vi "WPI_I2CVerifyString.vi"(8 "error in (no error)":errorcluster, 9 "Expected":string, 10 "Register Address":u8, 11 "I2CDevRef":T1={"DevStatus"={"status"=FALSE, "code"=0, "source"=""}, "Device Address"=0, "Handle"=0, "I2C Bus"=enum."Invalid"} {"Device Address" format="%.0x"}) -> (0 "error out":errorcluster, 3 "I2CDevRef":T1={"DevStatus"={"status"=FALSE, "code"=0, "source"=""}, "Device Address"=0, "Handle"=0, "I2C Bus"=enum."Invalid"} {"Device Address" format="%.0x"})   [LabVIEW 2017]
doc: "Reads consecutive registers from the I2C sensor you specify and compares the register strings to an expected value. This VI returns an error if the register strings do not match.\n\nThis software is licensed. Open the labview\\readme\\WPI Robotics Library Open Source License.txt file for more information."
uses:
  <vilib>/Rock Robotics/WPI/I2C/WPI_I2CDevRef.ctl
  <vilib>/Rock Robotics/SystemInterfaces/i2clib/i2c_bus.ctl
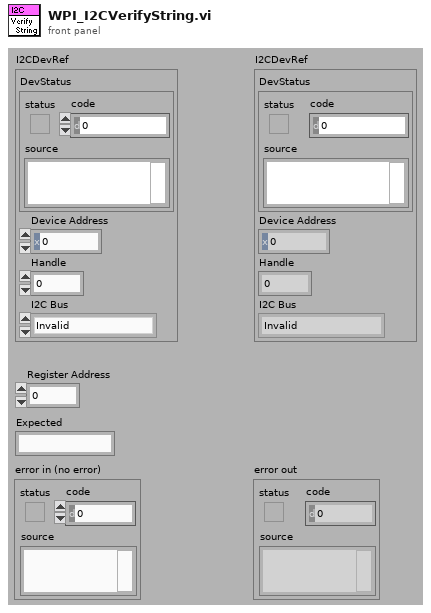
[diagram p1: front panel]
types:
  T1 = typedef "WPI_I2CDevRef.ctl" = cluster{"DevStatus":errorcluster, "Device Address":u8, "Handle":i32, "I2C Bus":T2}
  T2 = typedef "i2c_bus.ctl" = enum16{"I2C On-Board", "I2C MXP", "Invalid"}
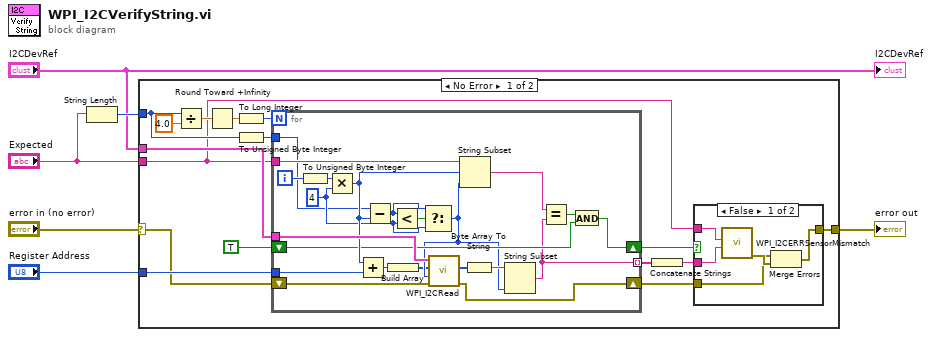
[diagram p0: block diagram]
diagram:
  n1 = String Length(string="Expected") -> (length=w5:i32)
  n2 = case shown="No Error" "error in (no error)" {
    selector: "error in (no error)" -> [w15 w51]
    tunnel: w5 -> [w11 _]
    tunnel: [w12 w51] -> w2
    tunnel: "Expected" -> [w7 _]
    tunnel: "I2CDevRef" -> [w17 _]
    tunnel: "Register Address" -> [w16 _]
    frame No Error {
      n3 = Divide(x=w11, y=4.0) -> (x/y=w21:dbl)
      n4 = Round Toward +Infinity(x=w21) -> (ceil(x): smallest int >= x=w20:dbl)
      n5 = To Long Integer(number=w20) -> (32bit integer=w19:i32)
      n6 = To Unsigned Byte Integer(number=w11) -> (unsigned 8bit integer=w10:u8)
      n7 = for {
        N: w19 -> [_]
        shift-right: [w36] -> w13
        shift-left: TRUE -> [w40]
        tunnel: w7 -> [w50]
        tunnel: w17 -> [w48]
        tunnel: w16 -> [w47]
        shift-right: [w33] -> w14
        shift-left: w15 -> [w38]
        tunnel: w10 -> [w37]
        tunnel: [w30] -> w9 mode=indexing
        i -> [w49]
        w41 = u8 4 ("length (rest)")
        n8 = To Unsigned Byte Integer(number=w49) -> (unsigned 8bit integer=w31:u8)
        n9 = Multiply(x=w31, y=w41) -> (x*y=w44:u8)
        n10 = Add(x=w44, y=w47) -> (x+y=w46:u8)
        n11 = Subtract(x=w37, y=w44) -> (x-y=w42:u8)
        n12 = Build Array(w46) -> (w29:u8[])
        n13 = Less?(x=w42, y=w41) -> (x < y?=w43:bool)
        n14 = Select(t=w42, s=w43, f=w41) -> (s? t:f=w32:u8)
        n15 = call <vilib>:"WPI_I2CRead.vi"("error in (no error)"=w38, "I2CBytesToRead"=w32, "I2CRegister"=w29, "I2CDevRef"=w48) -> ("error out"=w33:errorcluster, "Data Out"=w45:u8[])  [unwired: 6 out]
        n16 = String Subset(string=w50, offset (0)=w44, length (rest)=w32) -> (substring=w35:string)
        n17 = Byte Array To String(unsigned byte array=w45) -> (string=w34:string)
        n18 = String Subset(string=w34, length (rest)=w32) -> (substring=w30:string)  [unwired: 1 out]
        n19 = Equal?(x=w35, y=w30) -> (x = y?=w39:bool)
        n20 = And(x=w39, y=w40) -> (x .and. y?=w36:bool)
      }
      n21 = Concatenate Strings(w9) -> (w8:string)
      n22 = case shown="False" w13 {
        tunnel: w14 -> [w25 w28]
        tunnel: [w26 w28] -> w12
        tunnel: w8 -> [w24 _]
        tunnel: w7 -> [w23 _]
        frame False {
          n23 = call <vilib>:"WPI_I2CERRSensorMismatch.vi"("Read From Sensor"=w24, "Expected"=w23) -> ("ERRSensorMismatch"=w27:errorcluster)  [unwired: 9 out]
          n24 = Merge Errors(w25, w27) -> (w26:errorcluster)
        }
        frame True {
        }
      }
    }
    frame Error {
    }
  }
  "error out" <- w2
  "I2CDevRef" <- "I2CDevRef"
